vi "UI_updateWinnings.vi"(8 "error in (no error)":errorcluster, 10 "Winnings":dbl[](array[numeric]), 11 "Numeric Controls":refnum<vi>[](array[refnum])) -> (0 "error out":errorcluster)   [LabVIEW 2020]
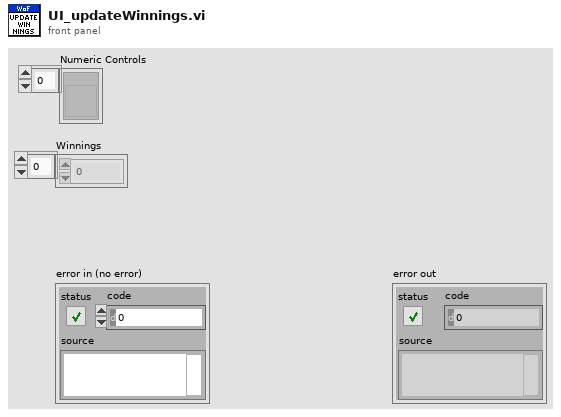
[diagram p1: front panel]
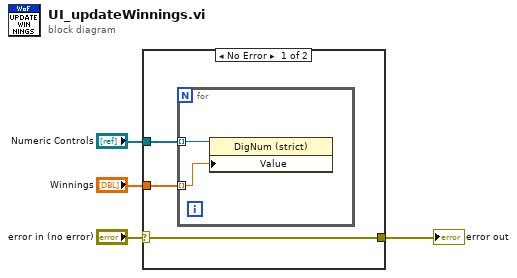
[diagram p0: block diagram]
diagram:
  n1 = case shown="No Error" "error in (no error)" {
    selector: "error in (no error)" -> [w6 w10]
    tunnel: "Winnings" -> [w7 _]
    tunnel: [w6 w10] -> w2
    tunnel: "Numeric Controls" -> [w5 _]
    frame No Error {
      n2 = for {
        tunnel: w7 -> [w8] mode=indexing
        tunnel: w5 -> [w9] mode=indexing
        n3 = property class="DigNum (strict)"(reference=w9, "Value"=w8) -> ()  [unwired: 1 in, 2 out]
      }
    }
    frame Error {
    }
  }
  "error out" <- w2
